vi "_USB_CAN_DEBUG_LOG_OUT_FUNC.vi"(11 "Info":string) -> ()   [LabVIEW 2011]
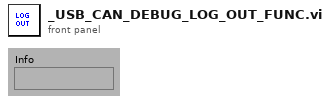
[diagram p1: front panel]
types:
  T1 = enum16{"open", "replace", "create", "open or create", "replace or create", "replace or create with confirmation"}
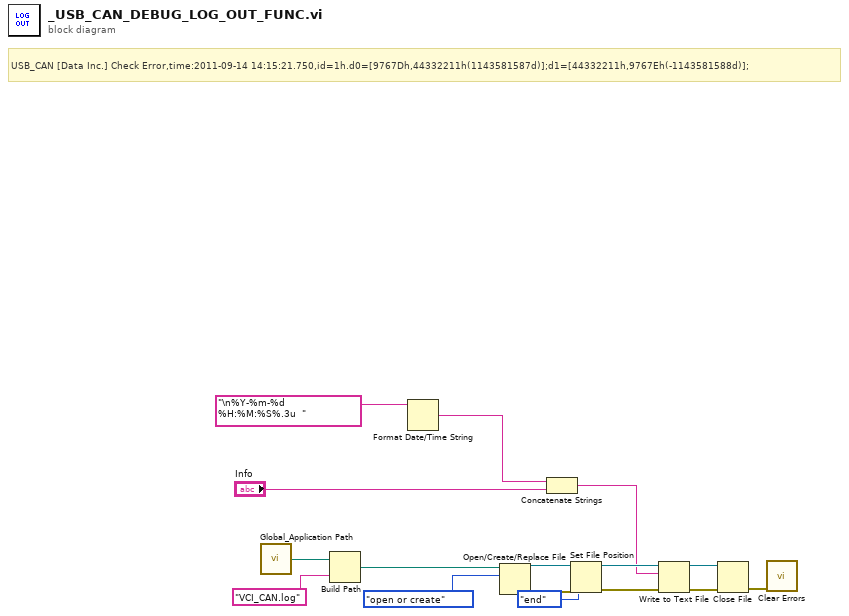
[diagram p0: block diagram]
diagram:
  # "USB_CAN [Data Inc.] Check Error,time:2011-09-14 14:15:21.750,id=1h.d0=[9767Dh,44332211h(1143581587d)];d1=[44332211h,9767Eh(-1143581588d)];"
  n1 = call "Global_Application Path.vi"() -> ("程序路径"=w4:path)  [unwired: 1 in]
  n2 = Build Path(base path=w4, name or relative path="VCI_CAN.log" ("名称或相对路径")) -> (appended path=w14:path)
  n3 = Format Date/Time String(time format string (%c)="\n%Y-%m-%d %H:%M:%S%.3u  " ("时间格式字符串(%c)")) -> (date/time string=w3:string)  [unwired: 2 in]
  n4 = Open/Create/Replace File(file path (use dialog)=w14, operation (0:open)=T1."open or create" ("操作(0:open)")) -> (refnum out=w12:refnum<file>, error out=w11:errorcluster)  [unwired: 4 in, 1 out]
  n5 = Concatenate Strings(w3, "Info") -> (w1:string)
  n6 = Set File Position(refnum=w12, from (0:start)=enum16{"start", "end", "current"}."end" ("自（0:起始）"), error in=w11) -> (refnum out=w9:refnum<file>, error out=w8:errorcluster)  [unwired: 1 in]
  n7 = Write to Text File(file (use dialog)=w9, text=w1, error in=w8) -> (refnum out=w6:refnum<file>, error out=w7:errorcluster)  [unwired: 1 in, 1 out]
  n8 = Close File(refnum=w6, error in=w7) -> (error out=w5:errorcluster)  [unwired: 1 out]
  n9 = call <vilib>:"Clear Errors.vi"("error in (no error)"=w5) -> ()  [unwired: 6 in, 1 out]
